vi "Update Waypoint Marker Image.vi"(8 "Error In":errorcluster, 10 "index":i32) -> (0 "error out":errorcluster)   [LabVIEW 2014]
uses:
  C:/Robotic Systems/Products/AgFalcon/Software/Ground Station/Data/Mapping DLL/GMap.NET.WindowsForms.dll
  Data/Mapping DLL/GMap.NET.WindowsForms.dll
  Reference/SubVI/Main Map Control Refernce.vi
  Reference/SubVI/GMap DLL Refernce.vi
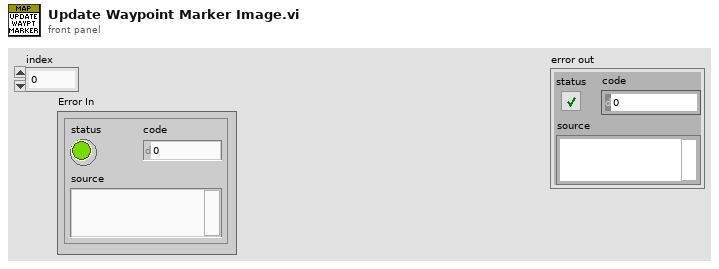
[diagram p1: front panel]
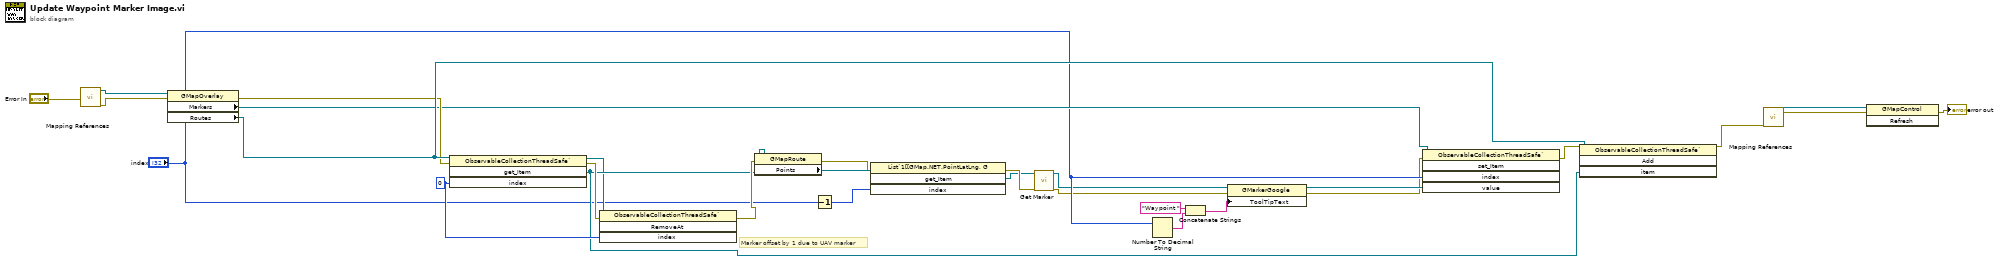
[diagram p0: block diagram]
diagram:
  w23 = 0 ("index")
  # "Marker offset by 1 due to UAV marker"
  n1 = call-poly "Mapping References.vi"("Error In"="Error In") -> ("Error Out"=w28:errorcluster, "Main Map Reference"=w29:refnum<k24>)  [unwired: 9 in]
  n2 = property class="GMapOverlay"(reference=w29, error in=w28) -> (error out=w14:errorcluster, "Markers"=w9:refnum<k24>, "Routes"=w15:refnum<k24>)  [unwired: 1 out]
  n3 = invoke class="ObservableCollectionThreadSafe`" method="get_Item"(reference=w15, error in=w14, "index"=w23) -> (reference out=w16:refnum<k24>, error out=w19:errorcluster, "get_Item"=w17:refnum<k24>)  [unwired: 1 in, 1 out]
  n4 = invoke class="ObservableCollectionThreadSafe`" method="RemoveAt"(reference=w16, error in=w19, "index"=w23) -> (error out=w22:errorcluster)  [unwired: 1 in, 3 out]
  n5 = property class="GMapRoute"(reference=w17, error in=w22) -> (error out=w13:errorcluster, "Points"=w26:refnum<k24>)  [unwired: 1 out]
  n6 = Decrement(x="index") -> (x-1=w25:i32)
  n7 = invoke class="List`1[[GMap.NET.PointLatLng, G" method="get_Item"(reference=w26, error in=w13, "index"=w25) -> (error out=w12:errorcluster, "get_Item"=w11:refnum<k24>)  [unwired: 1 in, 2 out]
  n8 = call "Get Marker.vi"("Error In"=w12, "Point"=w11) -> ("error out"=w4:errorcluster, "new reference"=w3:refnum<k24>)  [unwired: 8 in]
  n9 = Number To Decimal String(number="index") -> (decimal integer string=w8:string)  [unwired: 1 in]
  n10 = Concatenate Strings("Waypoint " ("string"), w8) -> (w6:string)
  n11 = property class="GMarkerGoogle"(reference=w3, error in=w4, "ToolTipText"=w6) -> (reference out=w2:refnum<k24>, error out=w1:errorcluster)
  n12 = invoke class="ObservableCollectionThreadSafe`" method="set_Item"(reference=w9, error in=w1, "index"="index", "value"=w2) -> (error out=w10:errorcluster)  [unwired: 1 in, 4 out]
  n13 = invoke class="ObservableCollectionThreadSafe`" method="Add"(reference=w15, error in=w10, "item"=w17) -> (error out=w18:errorcluster)  [unwired: 1 in, 3 out]
  n14 = call-poly "Mapping References.vi"("Error In"=w18) -> ("Error Out"=w21:errorcluster, "GMap DLL Reference"=w20:refnum<k24>)  [unwired: 9 in]
  n15 = invoke class="GMapControl" method="Refresh"(reference=w20, error in=w21) -> (error out=→"error out":errorcluster)  [unwired: 1 in, 2 out]
